vi "Test Process No Process Warnings Through Basic Lifecycle.vi"(8 "error in (no error)":errorcluster, 11 "Process Test In":refnum<class "Process Dev Test.lvclass">) -> (0 "error out":errorcluster, 3 "Process Test Out":refnum<class "Process Dev Test.lvclass">)   [LabVIEW 2020, in "Process Dev Test.lvclass"]
uses:
  Process Dev Test.lvclass
  C:/Program Files (x86)/National Instruments/LabVIEW 2020/vi.lib/Astemes/LUnit/Test Case.lvclass
  source/Framework Test Suite/Mock Error Handler/Mock Error Handler.lvclass
  C:/Git/triarc-framework/source/Framework/Error Handler Interface/Error Handler Interface.lvclass
  source/Framework/Process/Process.lvclass
  source/Framework/Process/Process.lvclass/Process.ctl
  <vilib>/Astemes/LUnit/Test Case.lvclass/Test Case.ctl
  <vilib>/Astemes/LUnit/LUnit Assertion Result.lvclass/LUnit Assertion Result.ctl
  <vilib>/Astemes/LUnit/LUnit Test Case Result.lvclass/LUnit Test Case Result.ctl
  <vilib>/Astemes/LUnit/LUnit Method Result.lvclass/LUnit Method Result.ctl
  source/Framework/Process/Protected/Messaging/Enqueue Message.vi
  source/Framework/Process/Public/Lifecycle/Get Lifecycle State.vi
  source/Framework/Process/Private/SubVIs/Wait for finish.vi
  source/Framework/Process/Private/SubVIs/Set Lifecycle State.vi
  <vilib>/Astemes/LUnit/Palette/Fail.vi
  <vilib>/Astemes/LUnit/Palette/Pass.vi
  <vilib>/Astemes/LUnit/Set Assertion Type.vi
  source/Framework/Process/Private/SubVIs/Handle Debug Data.vi
  <vilib>/Utility/error.llb/Clear Errors.vi
  <vilib>/Astemes/LUnit/Add test result.vi
  <vilib>/Astemes/LUnit/LUnit Write Passed.vi
  <vilib>/Astemes/LUnit/LUnit Write Message.vi
  <vilib>/Astemes/LUnit/LUnit Write Description.vi
  <vilib>/Astemes/LUnit/LUnit Write Assertion Type.vi
  source/Framework/Logging/Log Debug.vi
  <vilib>/AdvancedString/1D String Array to Delimited String.vi
  <vilib>/Utility/High Resolution Relative Seconds.vi
  <vilib>/Astemes/LUnit/LUnit Record Assertion Result.vi
  <vilib>/Astemes/LUnit/LUnit Aggregate Assertion Results.vi
  <vilib>/Astemes/LUnit/Assertion Result/LUnit Read Status.vi
  <vilib>/Astemes/LUnit/LUnit Read Message.vi
  <vilib>/Astemes/LUnit/LUnit Read Description.vi
  <vilib>/Astemes/LUnit/Method Result/LUnit Merge Status.vi
  <vilib>/Astemes/LUnit/LUnit Concatenate result strings.vi
  <vilib>/Utility/error.llb/Error Cluster From Error Code.vi
  source/Framework/Process/Public/Read Name.vi
  <vilib>/Astemes/LUnit/LUnit Assertion Result.lvclass
  <vilib>/Astemes/LUnit/Test Case.lvclass
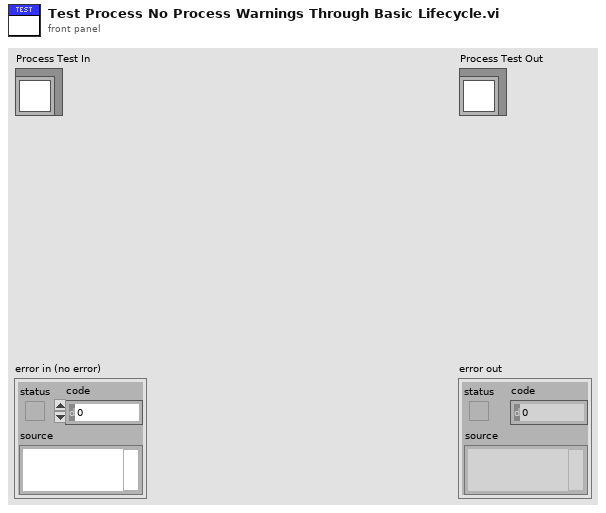
[diagram p1: front panel]
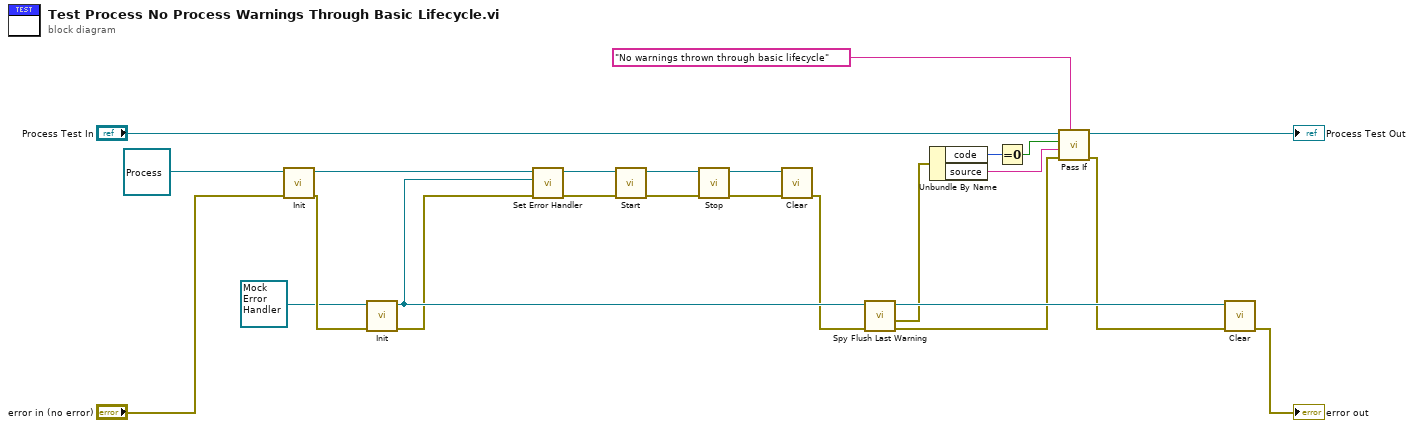
[diagram p0: block diagram]
diagram:
  n1 = call-dynamic "Init.vi"("error in (no error)"="error in (no error)", "Process In"=refnum<class "Process.lvclass"> refnum) -> ("error out"=w25:errorcluster, "Process Out"=w23:refnum<class "Process.lvclass">)  [unwired: 8 in]
  n2 = call-dynamic "Init.vi"("error in (no error)"=w25, "Mock Error Handler In"=refnum<class "Mock Error Handler.lvclass"> refnum ("Mock Error Handler.lvclass")) -> ("error out"=w15:errorcluster, "Mock Error Handler Out"=w16:refnum<class "Mock Error Handler.lvclass">)  [unwired: 8 in]
  n3 = call "Set Error Handler.vi"("error in (no error)"=w15, "Error Handler"=w16, "Process In"=w23) -> ("error out"=w21:errorcluster, "Process Out"=w22:refnum<class "Process.lvclass">)  [unwired: 7 in]
  n4 = call "Start.vi"("error in (no error)"=w21, "Process In"=w22) -> ("error out"=w19:errorcluster, "Process Out"=w20:refnum<class "Process.lvclass">)  [unwired: 7 in, 1 out]
  n5 = call "Stop.vi"("error in (no error)"=w19, "Process In"=w20) -> ("error out"=w17:errorcluster, "Process Out"=w18:refnum<class "Process.lvclass">)  [unwired: 7 in, 1 out]
  n6 = call-dynamic "Clear.vi"("error in (no error)"=w17, "Process In"=w18) -> ("error out"=w13:errorcluster)  [unwired: 9 in]
  n7 = call "Spy Flush Last Warning.vi"("error in (no error)"=w13, "Mock Error Handler In"=w16) -> ("error out"=w12:errorcluster, "Error"=w7:errorcluster, "Mock Error Handler Out"=w14:refnum<class "Mock Error Handler.lvclass">)  [unwired: 7 in]
  n8 = Unbundle By Name(w7) -> ("code"=w6:i32, "source"=w4:string)
  n9 = Equal To 0?(x=w6) -> (x = 0?=w5:bool)
  n10 = call <vilib>:"Pass If.vi"("Description"="No warnings thrown through basic lifecycle", "error in (no error)"=w12, "Message"=w4, "Pass?"=w5, "LUnit Test Case In"="Process Test In") -> ("error out"=w11:errorcluster, "LUnit Test Case Out"=→"Process Test Out":refnum<class "Process Dev Test.lvclass">)  [unwired: 5 in]
  n11 = call-dynamic "Clear.vi"("error in (no error)"=w11, "Mock Process In"=w14) -> ("error out"=→"error out":errorcluster)  [unwired: 9 in]
